vi "Toggle 1.vi"(1 "Input":bool) -> (0 "Output":bool)   [LabVIEW 2018]
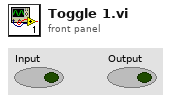
[diagram p1: front panel]
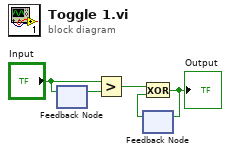
[diagram p0: block diagram]
diagram:
  n1 = feedback #1() -> (w4:bool)  [unwired: 1 in]
  n2 = feedback-in #1("Input") -> ()
  n3 = Greater?(x="Input", y=w4) -> (0:w2:bool)
  n4 = feedback #2() -> (w1:bool)  [unwired: 1 in]
  n5 = Exclusive Or(1:w1, 2:w2) -> (0:w5:bool)
  "Output" <- w5
  n6 = feedback-in #2(w5) -> ()
